vi "XY Graph Compute Thresholded Plot.vi"(6 "Threshold":dbl, 8 "Error In":errorcluster, 11 "Plot":T1) -> (0 "Error Out":errorcluster, 3 "Thresholded Plot":T1)   [LabVIEW 2021, in "XY Graph Add-Ons.lvlib"]
doc: "Set IRF values below threshold to zero."
uses:
  XY Graph Add-Ons.lvlib
  XY Graph Plot Data.ctl
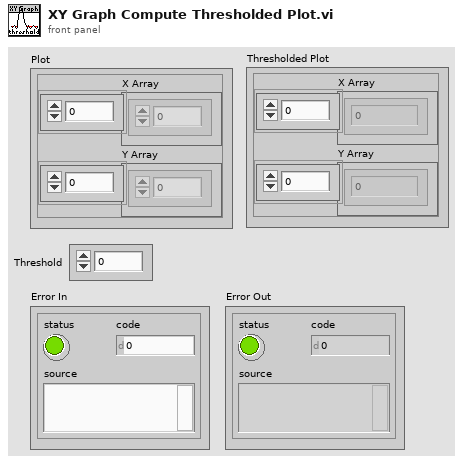
[diagram p1: front panel]
types:
  T1 = typedef "XY Graph Add-Ons.lvlib/XY Graph Plot Data.ctl" = cluster{"X Array":dbl[], "Y Array":dbl[]}
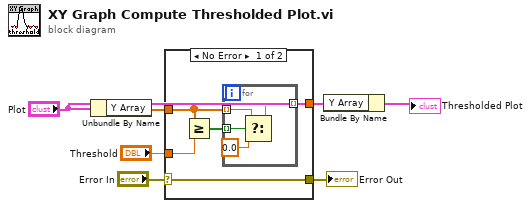
[diagram p0: block diagram]
diagram:
  n1 = Unbundle By Name("Plot") -> ("Y Array"=w4:dbl[])
  n2 = case shown="No Error" "Error In" {
    selector: "Error In" -> [w12 w18]
    tunnel: w4 -> [w9 w17]
    tunnel: [w12 w18] -> w7
    tunnel: [w8 w17] -> w2
    tunnel: "Threshold" -> [w11 _]
    frame No Error {
      n3 = Greater Or Equal?(x=w9, y=w11) -> (x >= y?=w10:bool[])
      n4 = for {
        tunnel: w10 -> [w16] mode=indexing
        tunnel: w9 -> [w15] mode=indexing
        tunnel: [w13] -> w8 mode=indexing
        n5 = Select(t=w15, s=w16, f=0.0) -> (s? t:f=w13:dbl)
      }
    }
    frame Error {
    }
  }
  "Error Out" <- w7
  n6 = Bundle By Name(cluster="Plot", "Y Array"=w2) -> (→"Thresholded Plot":T1)
